vi "GEA2 Read Message with Events.vi"(0 "GEA2 Event Registration":refnum<event-registration>, 11 "Error In":errorcluster) -> (4 "Coverted Data Out":T1 {"CRC" format="%04x"; "Length" format="%02x"; "Command" format="%02x"; "Destination" format="%02x"; "Source" format="%02x"}, 15 "Error Out":errorcluster)   [LabVIEW 2014, in "GEA2_Toolkit.lvlib"]
doc: "This VI accepts an event registration input. The input event is generated every time a message is present on the GEA2 bus. When an event is detected the event structure exectures and the output of this VI contains source and destination address as well as the command and data."
uses:
  library/GEA2_Toolkit.lvlib
  type defs/Data Out.ctl
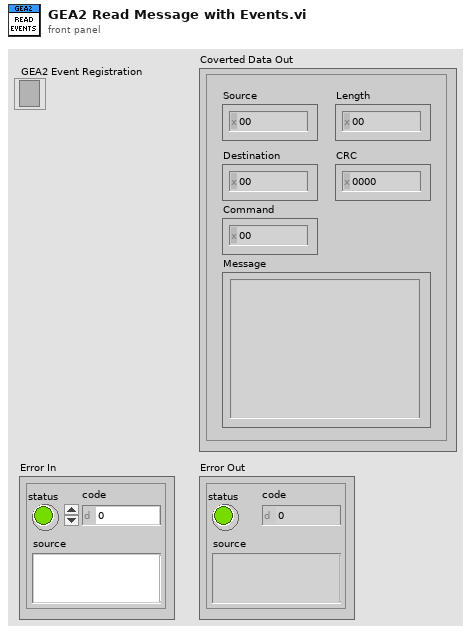
[diagram p1: front panel]
types:
  T1 = typedef "GEA2_Toolkit.lvlib/Data Out.ctl" = cluster{"Source":u8, "Destination":u8, "Command":u8, "Length":u8, "CRC":u16, "Message":string}
  T2 = typedef "eventsource.ctl" = u32
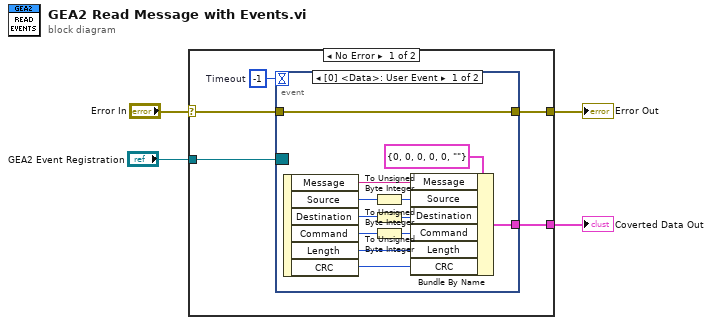
[diagram p0: block diagram]
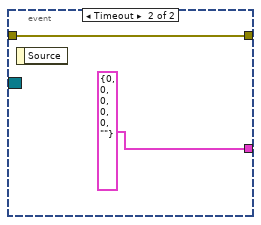
[diagram p2: hidden frame]
diagram:
  n1 = case shown="No Error" "Error In" {
    selector: "Error In" -> [w6 w24]
    tunnel: [w9 w24] -> w4
    tunnel: "GEA2 Event Registration" -> [w8 _]
    tunnel: [w5 _] -> w2
    frame No Error {
      w7 = -1  # Timeout
      n2 = event shown="[0] <Data>: User Event" {
        selector: w8 -> [_ _]
        dyn-events: _ -> [_ _]
        timeout: w7 -> [_ _]
        tunnel: w6 -> [w21 w23]
        tunnel: [w21 w23] -> w9
        tunnel: [w19 T1 {"Source"=0, "Destination"=0, "Command"=0, "Length"=0, "CRC"=0, "Message"=""} ("Coverted Data Out")] -> w5
        event User Event {
          n3 = event-data() -> ("Message"=w10:string, "Source"=w13:T2, "Destination"=w14:u8, "Command"=w15:u8, "Length"=w12:u8, "CRC"=w11:u16)  [unwired: 1 in]
          n4 = To Unsigned Byte Integer(number=w13) -> (unsigned 8bit integer=w17:u8)
          n5 = To Unsigned Byte Integer(number=w14) -> (unsigned 8bit integer=w18:u8)
          n6 = To Unsigned Byte Integer(number=w15) -> (unsigned 8bit integer=w16:u8)
          n7 = Bundle By Name(cluster=T1 {"Source"=0, "Destination"=0, "Command"=0, "Length"=0, "CRC"=0, "Message"=""} ("Coverted Data Out"), "Message"=w10, "Source"=w17, "Destination"=w18, "Command"=w16, "Length"=w12, "CRC"=w11) -> (w19:T1)
        }
        event Timeout {
          n8 = event-data() -> ()  [unwired: 1 in, 1 out]
        }
      }
    }
    frame Error {
    }
  }
  "Error Out" <- w4
  "Coverted Data Out" <- w2
